vi "Write Stop Refnum.vi"(8 "error in (no error)":errorcluster, 10 "Stop Refnum":refnum<vi>, 11 "New Session in":refnum<class "New Session.lvclass">) -> (0 "error out":errorcluster, 3 "New Session out":refnum<class "New Session.lvclass">)   [LabVIEW 2014, in "New Session Class.lvlib" / "New Session.lvclass"]
uses:
  New Session.lvclass
  New Session.lvclass/New Session.ctl
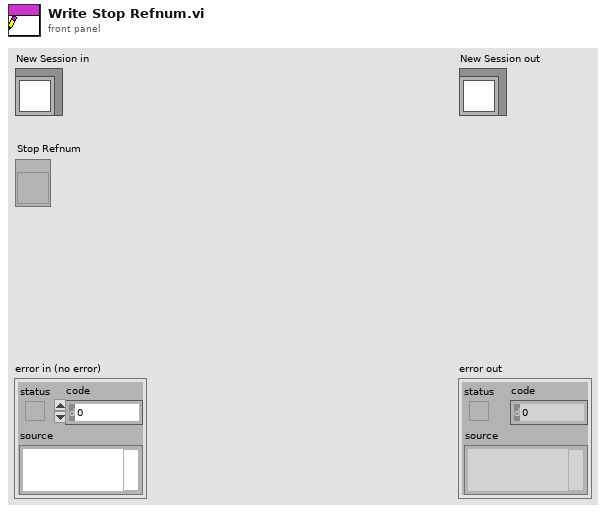
[diagram p1: front panel]
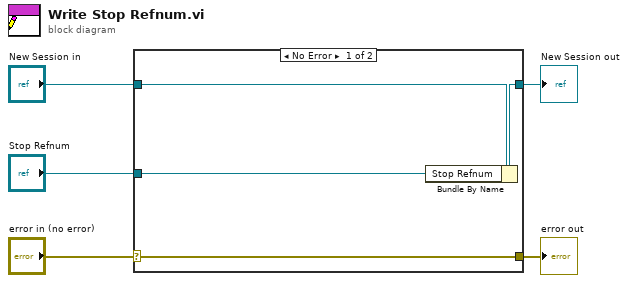
[diagram p0: block diagram]
diagram:
  n1 = case shown="No Error" "error in (no error)" {
    selector: "error in (no error)" -> [w9 w10]
    tunnel: [w9 w10] -> w4
    tunnel: [w7 w11] -> w2
    tunnel: "New Session in" -> [w8 w11]
    tunnel: "Stop Refnum" -> [w6 _]
    frame No Error {
      n2 = Bundle By Name(cluster=w8, "Stop Refnum"=w6) -> (w7:refnum<class "New Session.lvclass">)
    }
    frame Error {
    }
  }
  "error out" <- w4
  "New Session out" <- w2
